vi "LegalArmDistance.vi"(9 "WristAngle":dbl, 10 "ElbowAngle":dbl, 11 "ShoulderAngle":dbl) -> (2 "extensionLength":dbl, 3 "isBelowThirty":bool)   [LabVIEW 2018]
uses:
  <vilib>/Rock Robotics/WPI/MotorControl/WPI_MotorControlDeviceRef.ctl
  <vilib>/Rock Robotics/WPI/MotorControl/WPI_MotorControlType.ctl
  <vilib>/Rock Robotics/SystemInterfaces/DIO/FPGA_DIOPWMChannel.ctl
  <vilib>/Rock Robotics/WPI/PWM/WPI_PWMDeadband.ctl
  <vilib>/Rock Robotics/SystemInterfaces/DIO/FPGA_DIOChannel.ctl
  Arm Constants.vi
panel:
  in  "Shoulder":T1={"DeviceStatus"={"status"=FALSE, "code"=0, "source"=""}, "Type"=enum."PWM", "PWM"={"PWM Channel"=enum."PWM 1", "DeadBand"={"Name"="", "maxPositivePwm"=0, "minPositivePwm"=0, "centerPwm"=0, "maxNegativePwm"=0, "minNegativePwm"=0, "angularRange"=0}}, "CAN"={"Device Number"=0, "SetOutput VI Ref"=variant(enum8{"Percent VBus", "Current", "Speed", "Position", "Voltage"} enum."Percent VBus"), "GetOutput VI Ref"=variant(refnum<k1> refnum), "Enable VI Ref"=variant(dbl 12.0), "Disable VI Ref"=variant(enum8{"Percent VBus", "Speed", "Position", "Slave", "Unchanged / Invalid", "Voltage Compensation", "Current", "Motion Profile"} enum."Percent VBus"), "Data"=variant}, "Invert"=FALSE, "DIO PWM"={"PWM \"Enable\" Channel"=enum."Invalid", "DIOChannel"=enum."Invalid", "PWM Rate"=0.0}}
  in  "Elbow":T1={"DeviceStatus"={"status"=FALSE, "code"=0, "source"=""}, "Type"=enum."PWM", "PWM"={"PWM Channel"=enum."PWM 1", "DeadBand"={"Name"="", "maxPositivePwm"=0, "minPositivePwm"=0, "centerPwm"=0, "maxNegativePwm"=0, "minNegativePwm"=0, "angularRange"=0}}, "CAN"={"Device Number"=0, "SetOutput VI Ref"=variant(enum8{"Percent VBus", "Current", "Speed", "Position", "Voltage"} enum."Percent VBus"), "GetOutput VI Ref"=variant(refnum<k1> refnum), "Enable VI Ref"=variant(dbl 12.0), "Disable VI Ref"=variant(enum8{"Percent VBus", "Speed", "Position", "Slave", "Unchanged / Invalid", "Voltage Compensation", "Current", "Motion Profile"} enum."Percent VBus"), "Data"=variant}, "Invert"=FALSE, "DIO PWM"={"PWM \"Enable\" Channel"=enum."Invalid", "DIOChannel"=enum."Invalid", "PWM Rate"=0.0}}
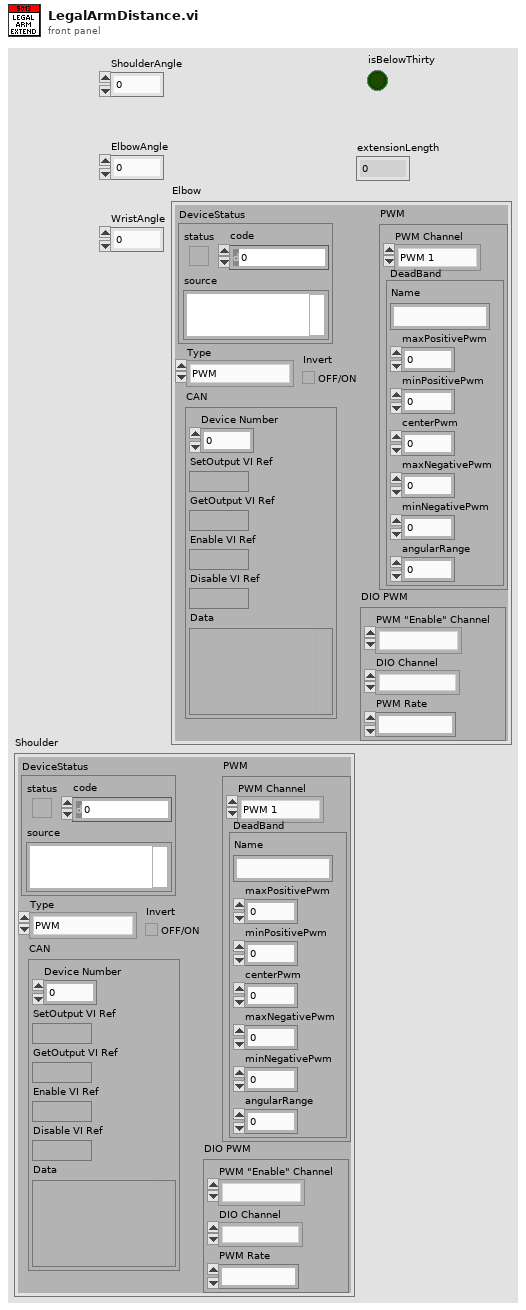
[diagram p1: front panel]
types:
  T1 = typedef "WPI_MotorControlDeviceRef.ctl" = cluster{"DeviceStatus":errorcluster, "Type":T2, "PWM":cluster{"PWM Channel":T3, "DeadBand":T4}, "CAN":cluster{"Device Number":u8, "SetOutput VI Ref":variant, "GetOutput VI Ref":variant, "Enable VI Ref":variant, "Disable VI Ref":variant, "Data":variant}, "Invert":bool, "DIO PWM":cluster{"PWM \"Enable\" Channel":T3, "DIOChannel":T5, "PWM Rate":dbl}}
  T2 = typedef "WPI_MotorControlType.ctl" = enum16{"PWM", "CAN", "DIO PWM"}
  T3 = typedef "FPGA_DIOPWMChannel.ctl" = enum8{"PWM 0", "PWM 1", "PWM 2", "PWM 3", "PWM 4", "PWM 5", "PWM 6", "PWM 7", "PWM 8", "PWM 9", "PWM MXP 0", "PWM MXP 1", "PWM MXP 2", "PWM MXP 3", "PWM MXP 4", "PWM MXP 5", "PWM MXP 6", "PWM MXP 7", "PWM MXP 8", "PWM MXP 9", "Invalid"}
  T4 = typedef "WPI_PWMDeadband.ctl" = cluster{"Name":string, "maxPositivePwm":i32, "minPositivePwm":i32, "centerPwm":i32, "maxNegativePwm":i32, "minNegativePwm":i32, "angularRange":u16}
  T5 = typedef "FPGA_DIOChannel.ctl" = enum8{"DIO 0", "DIO 1", "DIO 2", "DIO 3", "DIO 4", "DIO 5", "DIO 6", "DIO 7", "DIO 8", "DIO 9", "DIO MXP 0", "DIO MXP 1", "DIO MXP 2", "DIO MXP 3", "DIO MXP 4", "DIO MXP 5", "DIO MXP 6", "DIO MXP 7", "DIO MXP 8", "DIO MXP 9", "DIO MXP 10", "DIO MXP 11", "DIO MXP 12", "DIO MXP 13", "DIO MXP 14", "DIO MXP 15", "SPI Port CS1", "SPI Port CS2", "SPI Port CS3", "SPI Port MISO", "SPI Port MOSI", "Invalid"}
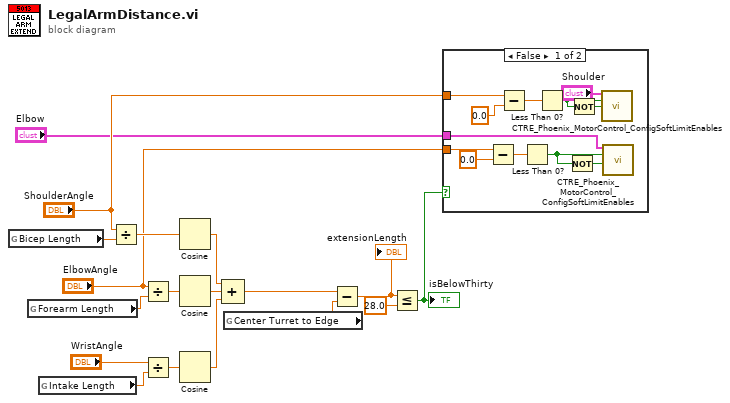
[diagram p0: block diagram]
diagram:
  n1 = global read "Arm Constants.vi" "Bicep Length"() -> (w5:dbl)
  n2 = global read "Arm Constants.vi" "Forearm Length"() -> (w6:dbl)
  n3 = global read "Arm Constants.vi" "Intake Length"() -> (w7:dbl)
  n4 = Divide(x="ShoulderAngle", y=w5) -> (x/y=w18:dbl)
  n5 = Divide(x="ElbowAngle", y=w6) -> (x/y=w17:dbl)
  n6 = Divide(x="WristAngle", y=w7) -> (x/y=w16:dbl)
  n7 = Cosine(x=w18) -> (cos(x)=w14:dbl)
  n8 = Cosine(x=w17) -> (cos(x)=w13:dbl)
  n9 = Cosine(x=w16) -> (cos(x)=w12:dbl)
  n10 = Compound Arithmetic op=ADD(w14, w13, w12) -> (w11:dbl)
  n11 = global read "Arm Constants.vi" "Center Turret to Edge"() -> (w8:dbl)
  n12 = Subtract(x=w11, y=w8) -> (x-y=w9:dbl)
  "extensionLength" <- w9
  n13 = Less Or Equal?(x=w9, y=28.0) -> (x <= y?=w3:bool)
  "isBelowThirty" <- w3
  n14 = case shown="False" w3 {
    tunnel: "ShoulderAngle" -> [w28 _]
    tunnel: "ElbowAngle" -> [w27 _]
    tunnel: "Elbow" -> [w19 _]
    frame False {
      n15 = Subtract(x=w27, y=0.0) -> (x-y=w23:dbl)
      n16 = Subtract(x=w28, y=0.0) -> (x-y=w29:dbl)
      n17 = Less Than 0?(x=w23) -> (x < 0?=w21:bool)
      n18 = Less Than 0?(x=w29) -> (x < 0?=w24:bool)
      n19 = Not(x=w21) -> (.not. x?=w22:bool)
      n20 = Not(x=w24) -> (.not. x?=w25:bool)
      n21 = call <vilib>:"CTRE_Phoenix_MotorControl_ConfigSoftLimitEnables.vi"("PhoenixMotorControlDevRef"="Shoulder", "Forward Soft Limit Enable"=w24, "Reverse Soft Limit Enable"=w25) -> ()  [unwired: 11 in, 2 out]
      n22 = call <vilib>:"CTRE_Phoenix_MotorControl_ConfigSoftLimitEnables.vi"("PhoenixMotorControlDevRef"=w19, "Forward Soft Limit Enable"=w21, "Reverse Soft Limit Enable"=w22) -> ()  [unwired: 11 in, 2 out]
    }
    frame True {
    }
  }
